vi "Get Versors.vi"(8 "error in (no error)":errorcluster, 11 "Angles":refnum<vi>) -> (0 "error out":errorcluster, 3 "Versor":cluster{"X":dbl, "Y":dbl, "Z":dbl})   [LabVIEW 2012, in "Targeting Unit.lvlib"]
uses:
  Targeting Unit.lvlib
panel:
  in  "Z direction":i8(ring)=-1 items=["Positive"=1, "Negative"=-1]
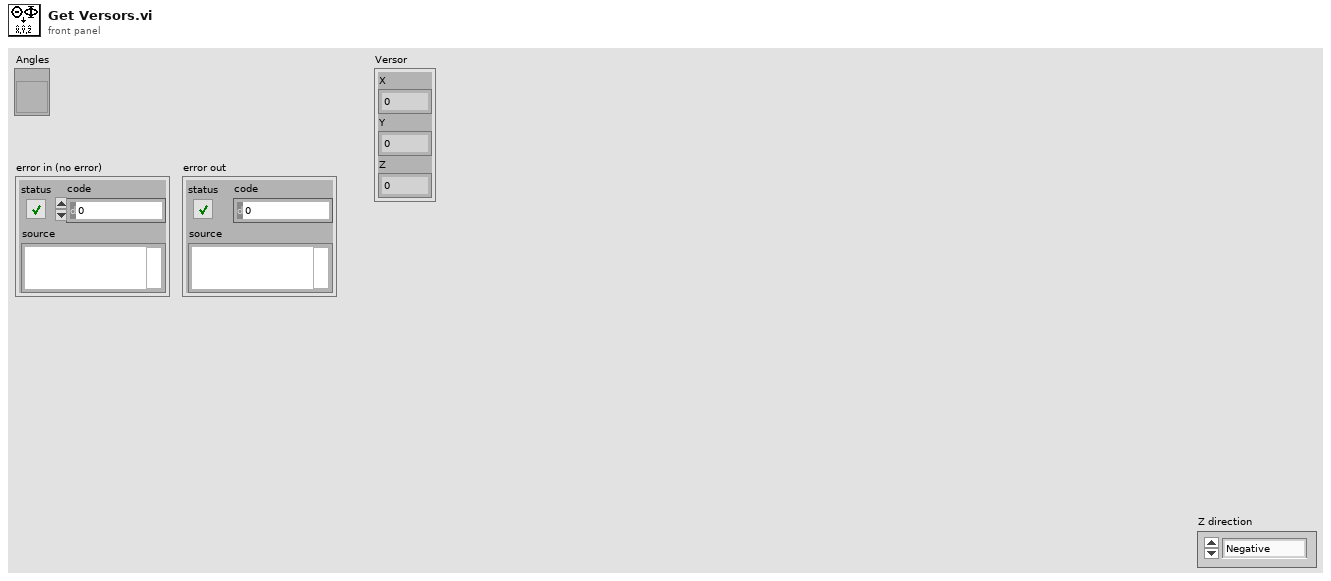
[diagram p1: front panel]
types:
  T1 = cluster{"X [um]":dbl, "Y [um]":dbl, "Z [um]":dbl}
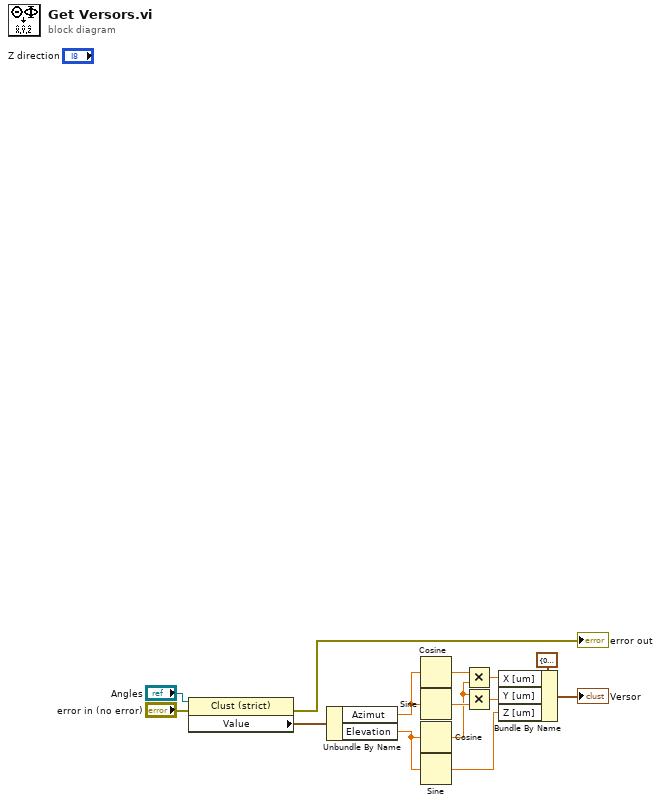
[diagram p0: block diagram]
diagram:
  n1 = property class="Clust (strict)"(reference="Angles", error in="error in (no error)") -> (error out=→"error out":errorcluster, "Value"=w7:cluster{"Azimut":dbl, "Elevation":dbl})  [unwired: 1 out]
  n2 = Unbundle By Name(w7) -> ("Azimut"=w8:dbl, "Elevation"=w5:dbl)
  n3 = Cosine(x=w8) -> (cos(x)=w11:dbl)
  n4 = Sine(x=w8) -> (sin(x)=w13:dbl)
  n5 = Cosine(x=w5) -> (cos(x)=w12:dbl)
  n6 = Sine(x=w5) -> (sin(x)=w6:dbl)
  n7 = Multiply(x=w11, y=w12) -> (x*y=w10:dbl)
  n8 = Multiply(x=w12, y=w13) -> (x*y=w9:dbl)
  n9 = Bundle By Name(cluster=T1 {"X [um]"=0.0, "Y [um]"=0.0, "Z [um]"=0.0} ("y"), "X [um]"=w10, "Y [um]"=w9, "Z [um]"=w6) -> (→"Versor":T1)
